vi "nirviRandomDataFpgaReadWriteTemplate.vi"(0 "Element in":variant, 1 "Timeout (ms)":i32, 3 "Fifo":T2={"displayName"="", "hardwareName"="", "dataType"=enum."I16", "elementTypeDescriptor"=variant, "terminalTypeDescriptor"=variant, "requestedNumberOfElements"=2, "memoryType"=enum."Look-Up Table", "arbitrationForInterfaceA"=enum."Arbitrate if Multiple Requestors Only", "numberOfElementsPerRead"=1, "arbitrationForInterfaceB"=enum."Always Arbitrate", "numberOfElementsPerWrite"=1, "VI_Defined"=FALSE, "type"=enum."Target-Scoped", "initializationParameters"={"initialized"=FALSE, "VI_Path"=path "", "initialData"=variant}, "disableOnOverflow/Underflow"=FALSE, "interfaceConfiguration"=enum."Read A-Write B", "controlLogic"=enum."Slice Fabric", "actualNumberOfElements"=1027, "dramSelection"="", "dramMaxOustandingRequests"=0, "dramIncludeByteEnables"=FALSE, "dramGrantTime"=0, "fullEmulation"=FALSE, "memoryInMultipleClockDomains"=FALSE, "memoryLatency"=1} {"memoryLatency" items=["0", "1", "2", "3"]}, 4 "Method":T1, 5 "error in (no error)":errorcluster, 6 "type":variant, 8 "In SCTL":bool, 9 "Input Valid?":bool, 11 "Ready for Output?":bool) -> (14 "element":variant, 15 "Timed out":bool, 16 "Ready for Input":bool, 17 "count":u32, 18 "Output Valid":bool, 19 "error out":errorcluster)   [LabVIEW 2020]
uses:
  <vilib>/rvi/DataTransferAndStorage/Container/Common/niFpgaContainerState.ctl
  <vilib>/rvi/DataTransferAndStorage/Container/Common/niFpgaDataTypeControl.ctl
  <vilib>/rvi/DataTransferAndStorage/Container/Common/niFpgaContainerImplementationControl.ctl
  <vilib>/rvi/DataTransferAndStorage/Container/Common/niFpgaContainerArbitrationOptionsControl.ctl
  <vilib>/rvi/DataTransferAndStorage/Container/Common/niFpgaTransferTypeControl.ctl
  <vilib>/rvi/DataTransferAndStorage/Container/Common/niFpgaContainerInitializationParameters.ctl
  <vilib>/rvi/Memory/Memory_Types/niFpgaMemoryInterfaceConfiguration.ctl
  <vilib>/rvi/FIFO/Fifo_Types/niFpgaFifoControlLogicControl.ctl
  <vilib>/rvi/DataTransferAndStorage/Container/Common/niFpgaContainerMemoryLatencyControl.ctl
  <vilib>/rvi/DataTransferAndStorage/Container/Common/niFpgaContainerMethod.ctl
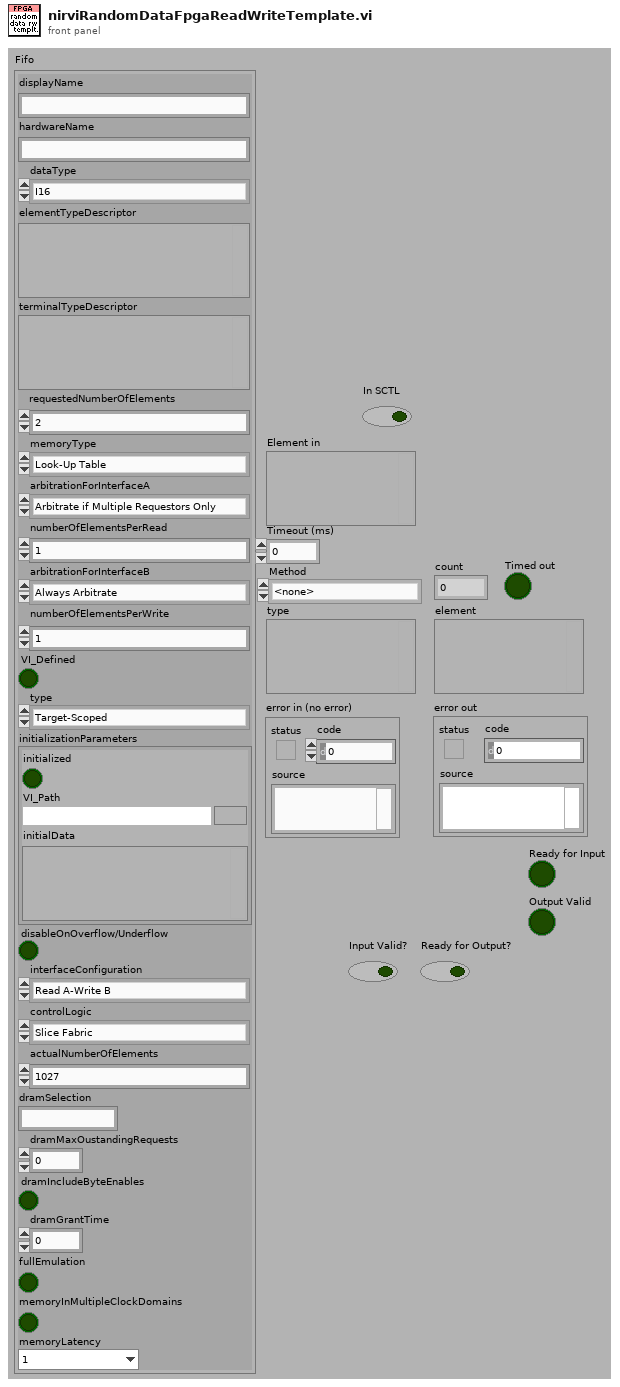
[diagram p1: front panel]
types:
  T1 = typedef "niFpgaContainerMethod.ctl" = enum16{"<none>", "write", "read", "clear", "getNumberOfElementsToWrite", "getNumberOfElementsToRead", "enable", "disable", "flushAndDisable", "getStreamState", "readA", "readB", "dramWrite", "dramWriteWithByteEnables", "dramRequestData", "dramRetrieveData", "readWithoutAcknowledge", "acknowledge", "writeUsingHandshaking", "readUsingHandshaking", "flush"}
  T2 = typedef "niFpgaContainerState.ctl" = cluster{"displayName":string, "hardwareName":string, "dataType":T3, "elementTypeDescriptor":variant, "terminalTypeDescriptor":variant, "requestedNumberOfElements":u32, "memoryType":T4, "arbitrationForInterfaceA":T5, "numberOfElementsPerRead":u32, "arbitrationForInterfaceB":T5, "numberOfElementsPerWrite":u32, "VI_Defined":bool, "type":T6, "initializationParameters":T7, "disableOnOverflow/Underflow":bool, "interfaceConfiguration":T8, "controlLogic":T9, "actualNumberOfElements":u32, "dramSelection":string, "dramMaxOustandingRequests":i32, "dramIncludeByteEnables":bool, "dramGrantTime":u32, "fullEmulation":bool, "memoryInMultipleClockDomains":bool, "memoryLatency":T10}
  T3 = typedef "niFpgaDataTypeControl.ctl" = enum32{"Boolean", "I8", "I16", "I32", "I64", "U8", "U16", "U32", "U64", "FXP", "CustomControl", "SGL"}
  T4 = typedef "niFpgaContainerImplementationControl.ctl" = enum16{"Flip-Flops", "Look-Up Table", "Block Memory", "DRAM", "UltraRAM"}
  T5 = typedef "niFpgaContainerArbitrationOptionsControl.ctl" = enum16{"Always Arbitrate", "Arbitrate if Multiple Requestors Only", "Never Arbitrate"}
  T6 = typedef "niFpgaTransferTypeControl.ctl" = enum16{"Target-Scoped", "Host to Target - DMA", "Target to Host - DMA", "Peer to Peer Reader", "Peer to Peer Writer", "Bidirectional"}
  T7 = typedef "niFpgaContainerInitializationParameters.ctl" = cluster{"initialized":bool, "VI_Path":path, "initialData":variant}
  T8 = typedef "niFpgaMemoryInterfaceConfiguration.ctl" = enum16{"Read A-Write B", "Read A-Read B"}
  T9 = typedef "niFpgaFifoControlLogicControl.ctl" = enum16{"Slice Fabric", "Target Optimal", "Built-in"}
  T10 = typedef "niFpgaContainerMemoryLatencyControl.ctl" = u16
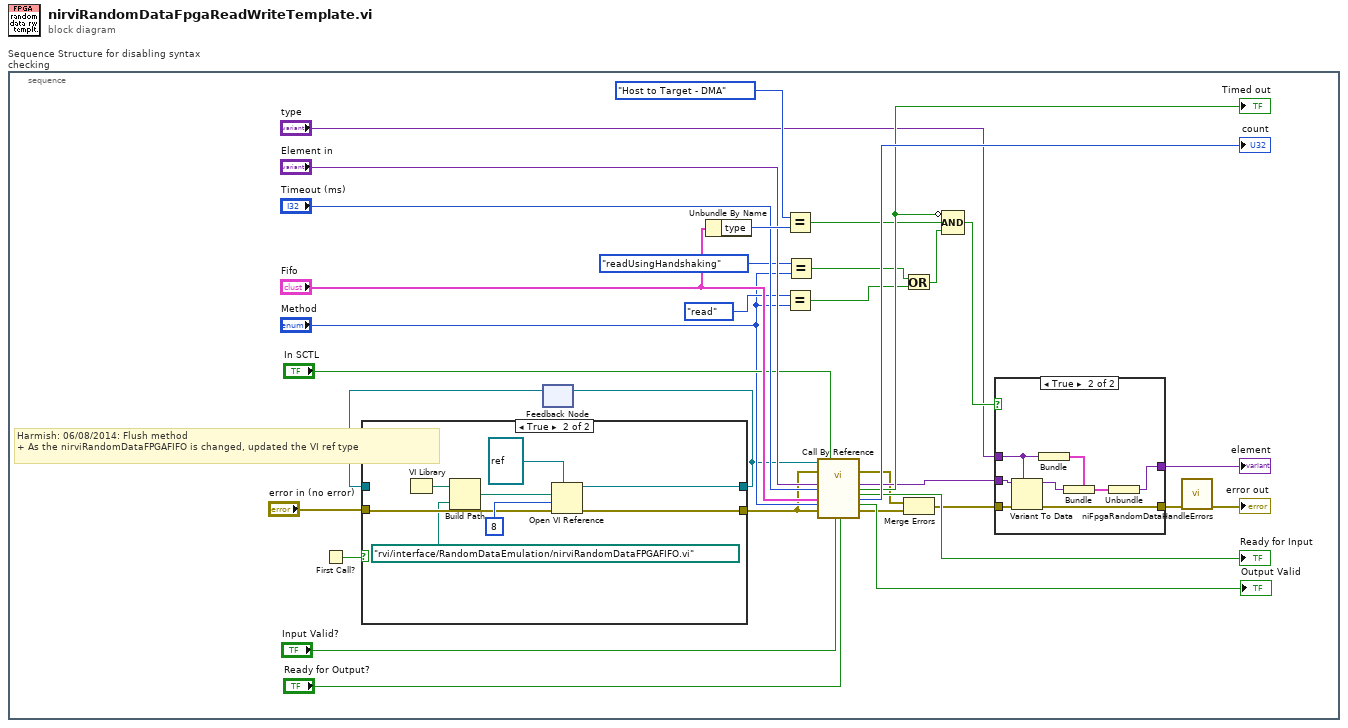
[diagram p0: block diagram]
diagram:
  n1 = stacked-sequence "Sequence Structure for disabling syntax checking" {
    frame #0 {
      # "Harmish: 06/08/2014: Flush method\n+ As the nirviRandomDataFPGAFIFO is changed, updated the VI ref type"
      n2 = First Call?() -> (First Call?: T/F=w5:bool)
      n3 = feedback #1() -> (w3:refnum<vi>)  [unwired: 1 in]
      n4 = case shown="True" w5 {
        tunnel: "error in (no error)" -> [w35 w40]
        tunnel: [w35 w39] -> w1
        tunnel: [w34 w38] -> w2
        tunnel: w3 -> [w34 _]
        frame False {
        }
        frame True {
          n5 = VI Library() -> (path=w41:path)
          n6 = Build Path(base path=w41, name or relative path=path "rvi/interface/RandomDataEmulation/nirviRandomDataFPGAFIFO.vi") -> (appended path=w42:path)
          n7 = Open VI Reference(type specifier VI Refnum (for type only)=refnum<vi> refnum, vi path=w42, options=8, error in (no error)=w40) -> (vi reference=w38:refnum<vi>, error out=w39:errorcluster)  [unwired: 2 in]
        }
      }
      n8 = feedback-in #1(w2) -> ()
      n9 = Unbundle By Name("Fifo") -> ("type"=w25:T6)
      n10 = Equal?(x=niFpgaTransferTypeControl."Host to Target - DMA" ("y"), y=w25) -> (x = y?=w26:bool)
      n11 = Equal?(x=niFpgaContainerMethod."read", y="Method") -> (x = y?=w18:bool)
      n12 = Equal?(x=niFpgaContainerMethod."readUsingHandshaking", y="Method") -> (x = y?=w17:bool)
      n13 = call-by-ref "?"(reference=w2, error in=w1, "element in"="Element in", "Timeout (ms)"="Timeout (ms)", "Fifo"="Fifo", "Method"="Method", 5:"error in (no error)"=w1, "In SCTL"="In SCTL", "Input Valid?"="Input Valid?", "Ready for Output?"="Ready for Output?") -> (error out=w8:errorcluster, "element out"=w24:variant, "Timed out"=w31:bool, "Ready for Input"=→"Ready for Input":bool, "count"=→"count":u32, "Output Valid"=→"Output Valid":bool, 19:"error out"=w7:errorcluster)  [unwired: 6 in, 1 out]
      "Timed out" <- w31
      n14 = Or(x=w17, y=w18) -> (x .or. y?=w19:bool)
      n15 = Merge Errors(w8, w7) -> (w6:errorcluster)
      n16 = Compound Arithmetic op=AND(invert w31, w26, w19) -> (w27:bool)
      n17 = case shown="True" w27 {
        tunnel: w6 -> [w44 w52]
        tunnel: "type" -> [_ w49]
        tunnel: w24 -> [_ w51]
        tunnel: [w44 w50] -> w28
        tunnel: [_ w45] -> w33
        frame False {
        }
        frame True {
          n18 = Variant To Data(error in=w52, type=w49, Variant=w51) -> (data=w47:variant, error out=w50:errorcluster)
          n19 = Bundle("type"=w49) -> (w48:cluster{"type":variant})  [unwired: 1 in]
          n20 = Bundle(cluster=w48, "type"=w47) -> (w46:cluster{"type":variant})
          n21 = Unbundle(w46) -> ("type"=w45:variant)
        }
      }
      "element" <- w33
      n22 = call <vilib>:"niFpgaRandomDataHandleErrors.vi"("error in"=w28) -> ("error out"=→"error out":errorcluster)  [unwired: 14 out]
    }
  }
